vi "Main_updated.vi"() -> ()   [LabVIEW 2016]
uses:
  Spreadsheet filling/Controls/Language Control.ctl
  types/Control_EXIT.ctl
  types/ctrlMainStates.ctl
  types/ctrlMainData.ctl
  Spreadsheet filling/Controls/Information_tab_type.ctl
  types/final data type.ctl
  <vilib>/Utility/miscctls.llb/LVPointTypeDef.ctl
  <vilib>/Utility/config.llb/Read Key (Boolean).vi
  <vilib>/Utility/config.llb/NI_LVConfig.lvlib
panel:
  in  "Exit":T1
  in  "Gas":bool
  out "Volume % Difference":dbl
  out "Progress":dbl(slide) scale=0.0..100.0
  in  "Software Version":string="1.09(US)"
  out "Sample in progress":bool
  out "Collect info done":bool
  in  "Sample method 2":u16(ring) items=["None", "Pulse Input", "Current Input", "Serial Input"]
  out "Mass % Difference":dbl
  in  "Sample \ninterval (S)":dbl=30.0
  in  "Language":T2
  in  "Collect info":bool
  in  "Export report":bool
  in  "Reset table":bool
  in  "Setpoint \n(kg/min)":dbl
  out "Data table":string[][](table)
  in  "Sample method 1":u16(ring) items=["None", "Pulse Input", "Current Input", "Serial Input"]
  in  "Begin pulse sample":bool
  in  "Transfer Data":bool
  in  "Run #":u16
  # "Flow Lifecycle Calibration Services"
  # "Mass\n(UUT)"
  # "Mass\n(Master)"
  # "Mass \n% diff"
  # "Volume\n(UUT)"
  # "Volume\n(Master)"
  # "Setpoint"
  # "Run"
  # "Select an input type"
  # "Select an input type"
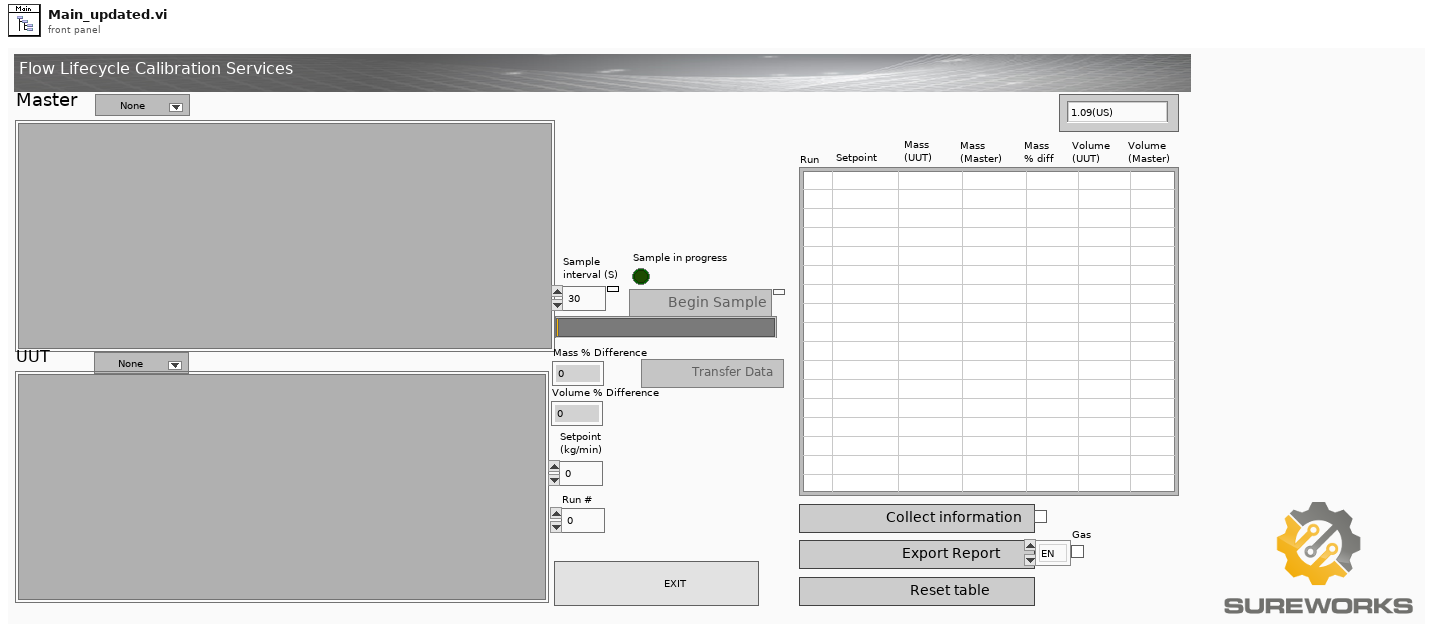
[diagram p1: front panel]
types:
  T1 = typedef "Control_EXIT.ctl" = bool
  T2 = typedef "Language Control.ctl" = enum16{"EN", "ES", "FR", "RU"}
  T3 = typedef "ctrlMainData.ctl" = cluster{"HART ports":refnum<visa-resource-name>[], "485 ports":refnum<visa-resource-name>[], "Byte order":enum16{"0-1-2-3", "2-3-0-1", "1-0-3-2", "3-2-1-0"}, "Information":T4, "Base path":path, "MasterVIRef":refnum<vi>, "UUTVIRef":refnum<vi>, "VIList":string[], "Collect info done":bool, "LeaveExcelOpen":bool, "Sample complete":bool, "Final data":T5, "StartTime":timestamp}
  T4 = typedef "Information_tab_type.ctl" = cluster{"Test Date and Time, 1":string, "Test Comments,3":string, "Sensor Serial Number,6":string, "Sensor Model,7":string, "Size,8":string, "Material,9":string, "Press rating, 10":string, "Temp rating, 11":string, "FCF, 14":string, "D1, 15":string, "D2, 16":string, "K1, 17":string, "K2, 18":string, "FD, 19":string, "Density Temp Coeff, 20":string, "Transmitter Serial Number,23":string, "Transmitter Model Number,24":string, "Mass Flow Units, 25":string, "Density Units, 26":string, "Temperature Units, 27":string, "Mass Flow Cutoff, 28":string, "Mass Flow Damping, 29":string, "Flow Direction, 30":string, "Frequency Flow Rate, 31":string, "Frequency Span, 32":string, "Flow Accuracy, 35":string, "Flow Repeatability, 36":string, "Zero Stability, 37":string, "Density Accuracy, 38":string, "Density Repeatability, 39":string, "Nomincal Flow Rate, 41":string, "Meter Zero, 43":string, "Status, 45":string, "Customer name, 46":string, "Customer address, 47":string, "Sales order number, 48":string, "Technician Name, 49":string, "ref meter, 50":string, "product code,51":string, "fluid,52":string, "fluid temp,53":string}
  T5 = typedef "final data type.ctl" = cluster{"Master final data":cluster{"Mass total":dbl, "Volume total":dbl, "Density mean":dbl}, "UUT final data":cluster{"Mass total":dbl, "Volume total":dbl, "Density mean":dbl}}
  T6 = typedef "ctrlMainStates.ctl" = enum16{"WaitforEvents", "Init", "Close", "SampleStarted", "SampleComplete", "TransferData", "UpdateSampleMethod1", "UpdateSampleMethod2", "ExportReport", "CollectInfo", "ResetTable", "BeginPulseSample"}
  T7 = enum8{"Enabled", "Disabled", "Disabled and Grayed Out"}
  T8 = typedef "LVPointTypeDef.ctl" = cluster{"Horizontal":i16, "Vertical":i16}
  T9 = typedef "NI_LVConfig.lvlib/Config Data RefNum.ctl" = refnum<k1>
  T10 = enum16{"0-1-2-3", "2-3-0-1", "1-0-3-2", "3-2-1-0"}
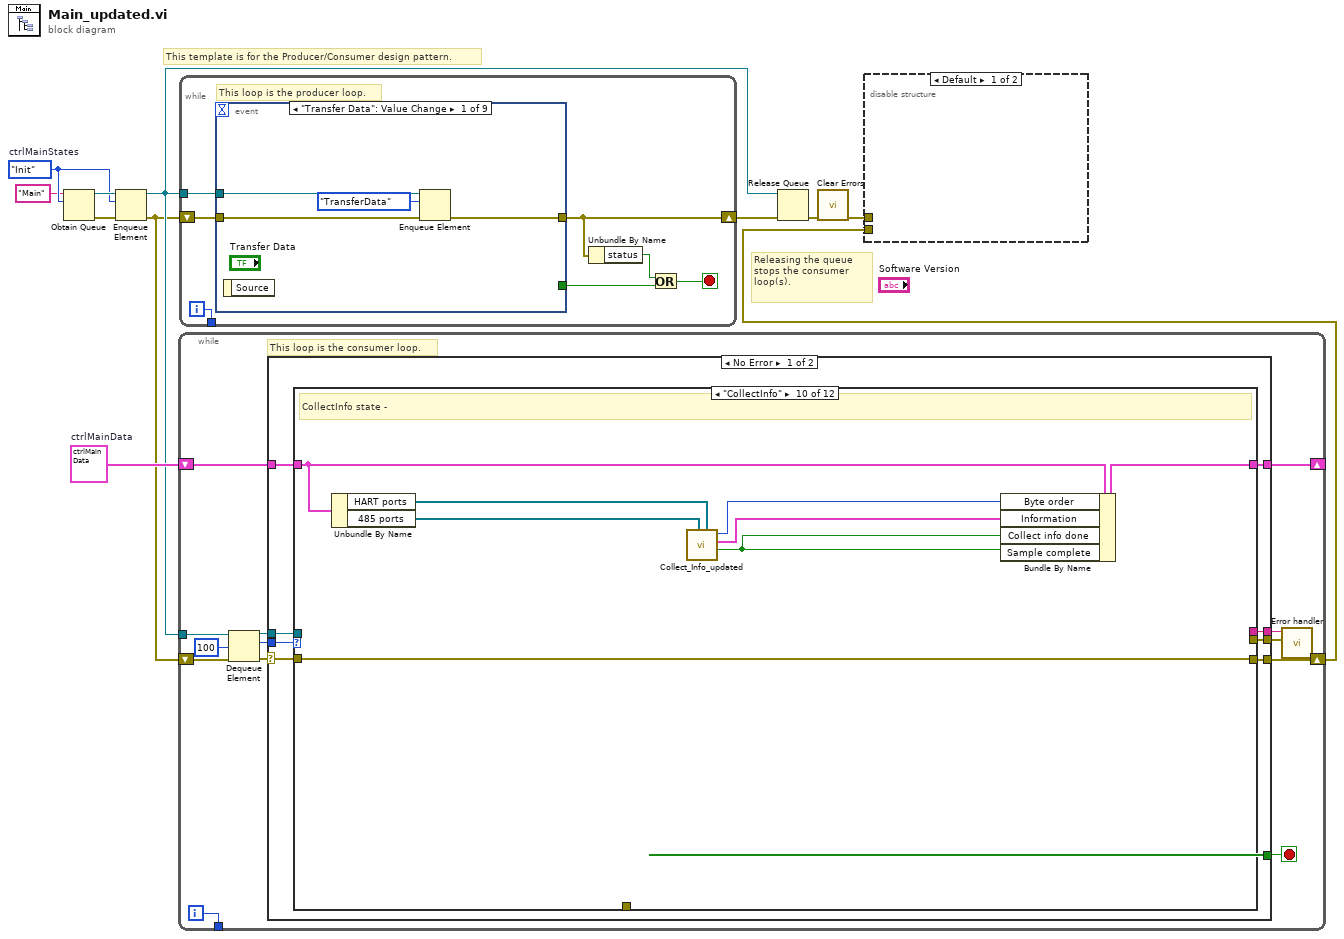
[diagram p0: block diagram]
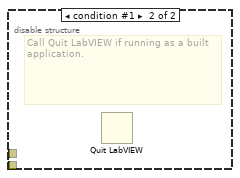
[diagram p2: hidden frame]
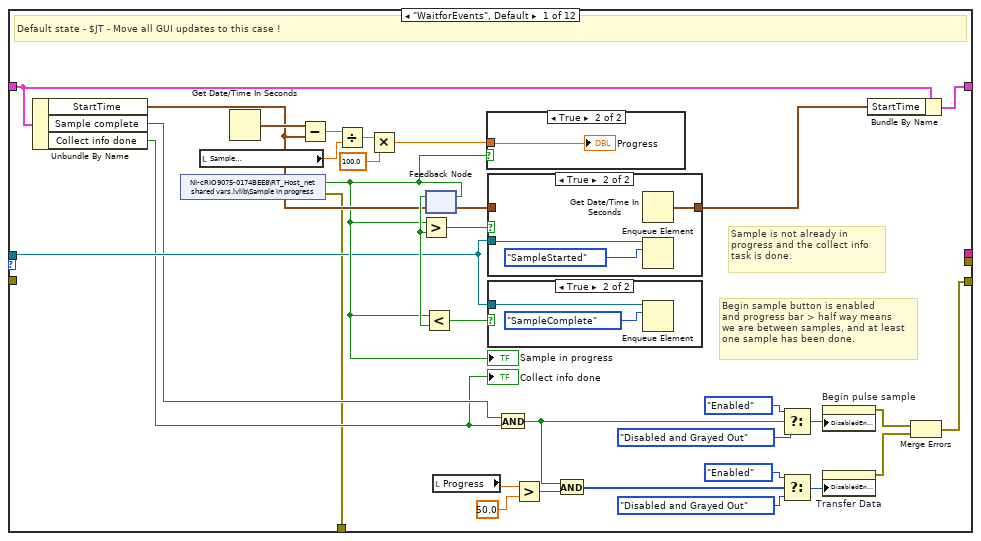
[diagram p3: hidden frame]
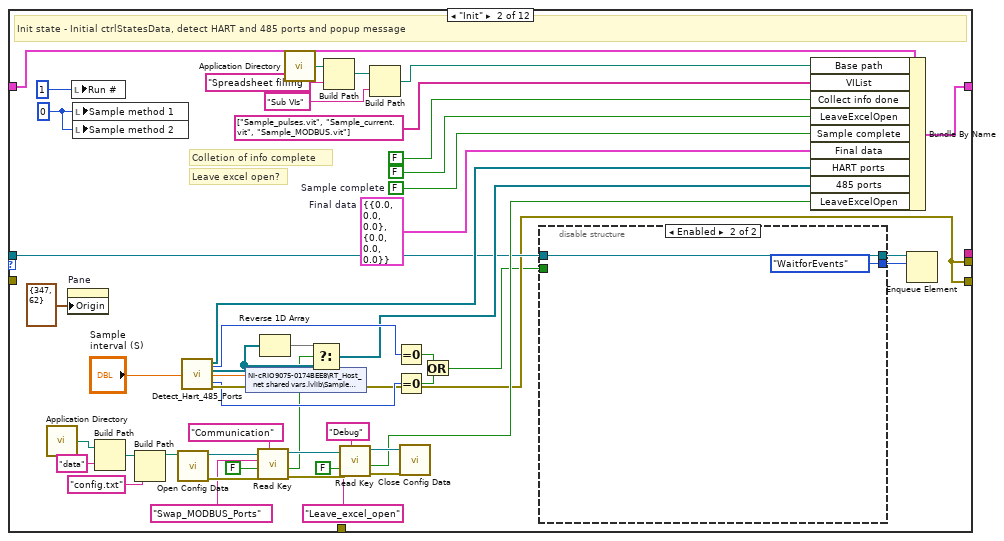
[diagram p7: hidden frame]
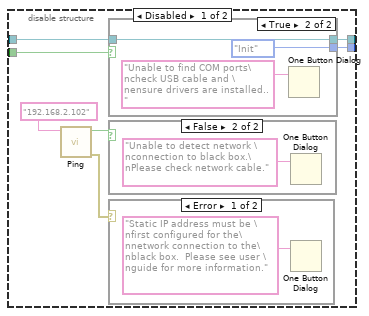
[diagram p8: hidden frame]
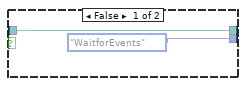
[diagram p9: hidden frame]
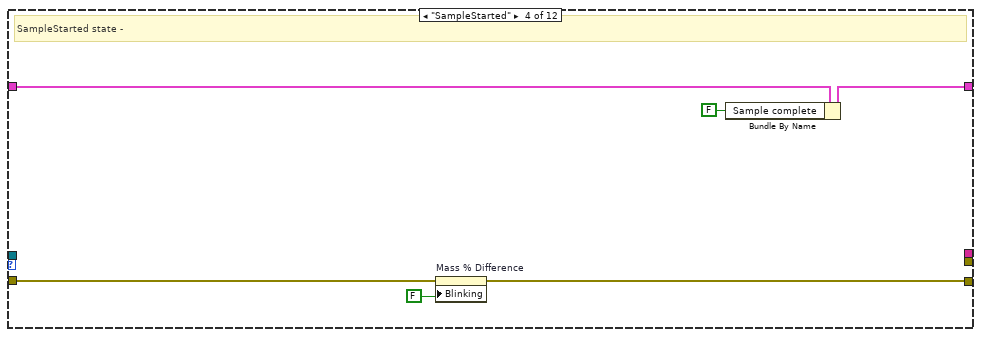
[diagram p13: hidden frame]
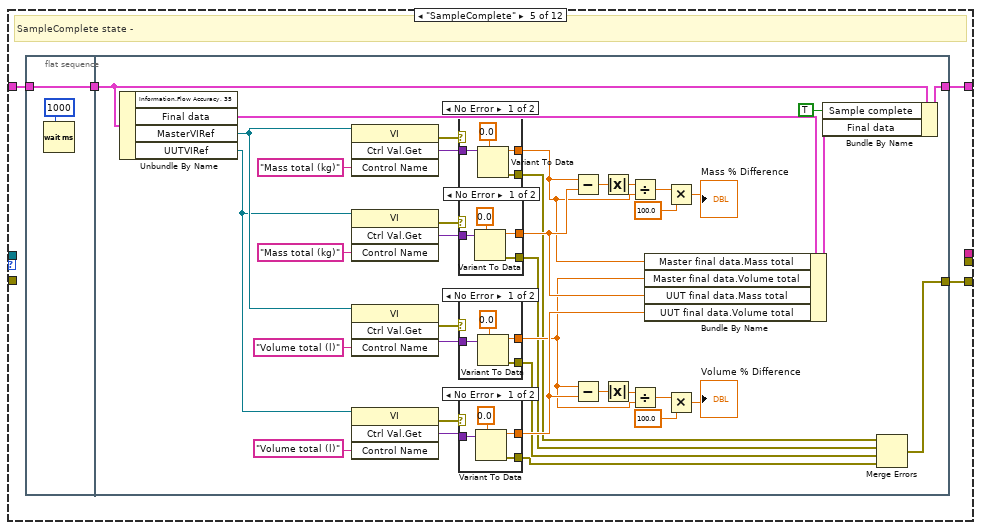
[diagram p14: hidden frame]
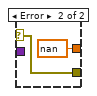
[diagram p15: hidden frame]
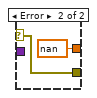
[diagram p16: hidden frame]
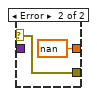
[diagram p17: hidden frame]
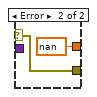
[diagram p18: hidden frame]
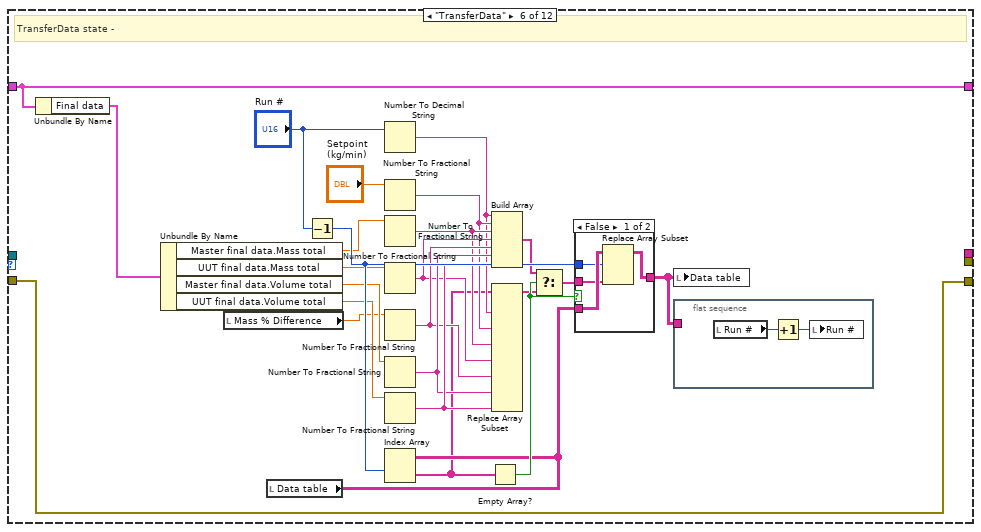
[diagram p19: hidden frame]
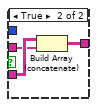
[diagram p20: hidden frame]
diagram:
  w11 = T3 {"HART ports"=[], "485 ports"=[], "Byte order"=enum."0-1-2-3", "Information"={"Test Date and Time, 1"="", "Test Comments,3"="", "Sensor Serial Number,6"="", "Sensor Model,7"="", "Size,8"="", "Material,9"="", "Press rating, 10"="", "Temp rating, 11"="", "FCF, 14"="", "D1, 15"="", "D2, 16"="", "K1, 17"="", "K2, 18"="", "FD, 19"="", "Density Temp Coeff, 20"="", "Transmitter Serial Number,23"="", "Transmitter Model Number,24"="", "Mass Flow Units, 25"="", "Density Units, 26"="", "Temperature Units, 27"="", "Mass Flow Cutoff, 28"="", "Mass Flow Damping, 29"="", "Flow Direction, 30"="", "Frequency Flow Rate, 31"="", "Frequency Span, 32"="", "Flow Accuracy, 35"="", "Flow Repeatability, 36"="", "Zero Stability, 37"="", "Density Accuracy, 38"="", "Density Repeatability, 39"="", "Nomincal Flow Rate, 41"="", "Meter Zero, 43"="", "Status, 45"="", "Customer name, 46"="", "Customer address, 47"="", "Sales order number, 48"="", "Technician Name, 49"="", "ref meter, 50"="", "product code,51"="", "fluid,52"="", "fluid temp,53"=""}, "Base path"=path "", "MasterVIRef"=refnum, "UUTVIRef"=refnum, "VIList"=[], "Collect info done"=FALSE, "LeaveExcelOpen"=FALSE, "Sample complete"=FALSE, "Final data"={"Master final data"={"Mass total"=0.0, "Volume total"=0.0, "Density mean"=0.0}, "UUT final data"={"Mass total"=0.0, "Volume total"=0.0, "Density mean"=0.0}}, "StartTime"=timestamp(0 s since 1904-01-01)}  # ctrlMainData
  w8 = ctrlMainStates."Init"  # ctrlMainStates
  # "This template is for the Producer/Consumer design pattern."
  # "Releasing the queue stops the consumer loop(s)."
  n1 = Obtain Queue(name (unnamed)="Main", element data type=w8) -> (queue out=w10:refnum<queue>, error out=w4:errorcluster)  [unwired: 3 in, 1 out]
  n2 = Enqueue Element(queue=w10, element=w8, error in (no error)=w4) -> (queue out=w9:refnum<queue>, error out=w3:errorcluster)  [unwired: 1 in, 1 out]
  n3 = while {
    tunnel: w9 -> [w24]
    shift-right: [w18] -> _
    shift-left: w11 -> [w20]
    shift-right: [w13] -> w1
    shift-left: w3 -> [w15]
    tunnel: [w12] -> _
    i -> [w12]
    stop <- w21 stop-if-true
    # "This loop is the consumer loop."
    n4 = Dequeue Element(queue=w24, timeout in ms (-1)=100, error in (no error)=w15) -> (queue out=w17:refnum<queue>, element=w22:T6, error out=w23:errorcluster)  [unwired: 1 out]
    n5 = case shown="No Error" w23 {
      selector: w23 -> [w25 w320]
      tunnel: w22 -> [w30 _]
      tunnel: [_ TRUE] -> w21
      tunnel: w20 -> [w31 w321]
      tunnel: [w32 w321] -> w18
      tunnel: w17 -> [w29 _]
      tunnel: [w28 _] -> w14
      tunnel: [w27 _] -> w16
      tunnel: [w26 w319] -> w13
      frame No Error {
        n6 = case shown="\"CollectInfo\"" w30 {
          tunnel: [w55 w109 w138 w141 w148 w215 w250 w263 w281 w299 w305 w318] -> w32
          tunnel: w31 -> [w53 w110 w138 w143 w147 w215 w248 w264 w281 w300 w307 w318]
          tunnel: w29 -> [w50 w77 _ _ _ _ _ _ _ _ _ _]
          tunnel: [_ w74 _ _ _ _ w247 w262 w277 _ _ _] -> w28
          tunnel: [_ _ _ _ _ _ _ _ "Error in PDF path.  Please check that the data output folder exists." ("Error reason") _ _ _] -> w27
          tunnel: [w34 w74 w137 w139 w145 w213 w247 w262 w277 w295 w303 w317] -> w26
          tunnel: w25 -> [_ _ w137 w140 _ w213 _ _ _ w295 w303 w317]
          tunnel: [w33 _ _ _ _ _ _ _ _ _ _ _] -> _
          frame "WaitforEvents", Default {
            # "Begin sample button is enabled\nand progress bar > half way means \nwe are between samples, and at least\none sample has been done."
            # "Sample is not already in\nprogress and the collect info \ntask is done."
            # "Default state - $JT - Move all GUI updates to this case !"
            n7 = Unbundle By Name(w53) -> ("StartTime"=w52:timestamp, "Sample complete"=w46:bool, "Collect info done"=w37:bool)
            "Collect info done" <- w37
            n8 = shared-variable "NI-cRIO9075-0174BEE8\\RT_Host_net shared vars.lvlib\\Sample in progress"() -> (w51:bool, error out=w33:errorcluster)  [unwired: 1 in]
            "Sample in progress" <- w51
            n9 = local read "Sample \ninterval (S)"() -> (w61:dbl)
            n10 = Get Date/Time In Seconds() -> (seconds since 1Jan1904=w59:timestamp)
            n11 = Subtract(x=w59, y=w52) -> (x-y=w60:dbl)
            n12 = Divide(x=w60, y=w61) -> (x/y=w62:dbl)
            n13 = Multiply(x=w62, y=100.0) -> (x*y=w64:dbl)
            n14 = feedback #1() -> (w57:bool)  [unwired: 1 in]
            n15 = Greater?(x=w51, y=w57) -> (0:w56:bool)
            n16 = Less?(x=w51, y=w57) -> (x < y?=w58:bool)
            n17 = feedback-in #1(w51) -> ()
            n18 = local read "Progress"() -> (w41:dbl)
            n19 = case shown="True" w51 {
              tunnel: w64 -> [_ w65]
              frame False {
              }
              frame True {
                "Progress" <- w65
              }
            }
            n20 = case shown="True" w56 {
              tunnel: w50 -> [_ w69]
              tunnel: [w68 w71] -> w54
              tunnel: w52 -> [w68 _]
              frame False {
              }
              frame True {
                n21 = Get Date/Time In Seconds() -> (seconds since 1Jan1904=w71:timestamp)
                n22 = Enqueue Element(queue=w69, element=ctrlMainStates."SampleStarted" ("ctrlStates")) -> ()  [unwired: 2 in, 3 out]
              }
            }
            n23 = case shown="True" w58 {
              tunnel: w50 -> [_ w67]
              frame False {
              }
              frame True {
                n24 = Enqueue Element(queue=w67, element=ctrlMainStates."SampleComplete" ("ctrlStates")) -> ()  [unwired: 2 in, 3 out]
              }
            }
            n25 = And(x=w46, y=w37) -> (x .and. y?=w38:bool)
            n26 = Greater?(x=w41, y=50.0) -> (0:w39:bool)
            n27 = And(x=w38, y=w39) -> (x .and. y?=w42:bool)
            n28 = Select(t=T7."Enabled" ("Disabled"), s=w38, f=T7."Disabled and Grayed Out" ("Disabled")) -> (s? t:f=w47:T7)
            n29 = Select(t=T7."Enabled" ("Disabled"), s=w42, f=T7."Disabled and Grayed Out" ("Disabled")) -> (s? t:f=w43:T7)
            n30 = property on="Begin pulse sample" class="Bool (strict)"("DisabledEnum"=w47) -> (error out=w36:errorcluster)  [unwired: 2 in, 1 out]
            n31 = property on="Transfer Data" class="Bool"("DisabledEnum"=w43) -> (error out=w35:errorcluster)  [unwired: 2 in, 1 out]
            n32 = Bundle By Name(cluster=w53, "StartTime"=w54) -> (w55:T3)
            n33 = Merge Errors(w36, w35) -> (w34:errorcluster)
          }
          frame "Init" {
            w78 = T5 {"Master final data"={"Mass total"=0.0, "Volume total"=0.0, "Density mean"=0.0}, "UUT final data"={"Mass total"=0.0, "Volume total"=0.0, "Density mean"=0.0}}  # Final data
            w79 = FALSE  # Sample complete
            w120 = u16 0 ("Run")
            # "Leave excel open?"
            # "Colletion of info complete"
            # "Init state - Initial ctrlStatesData, detect HART and 485 ports and popup message"
            n34 = call <vilib>:"Application Directory.vi"() -> ("Application Directory"=w104:path)
            n35 = property on="Pane" class="Pane"("Origin"=T8 {"Horizontal"=347, "Vertical"=62}) -> ()  [unwired: 2 in, 2 out]
            n36 = local write "Run #"(u16 1 ("Run #")) -> ()
            n37 = local write "Sample method 1"(w120) -> ()
            n38 = local write "Sample method 2"(w120) -> ()
            n39 = Build Path(base path=w104, name or relative path="data") -> (appended path=w103:path)
            n40 = Build Path(base path=w103, name or relative path="config.txt") -> (appended path=w106:path)
            n41 = call <vilib>:"Open Config Data.vi"("configuration file path"=w106) -> ("error out"=w100:errorcluster, "refnum"=w101:T9)  [unwired: 8 in, 1 out]
            n42 = call "Detect_Hart_485_Ports.vi"() -> ("error out"=w118:errorcluster, "485 Ports"=w112:refnum<visa-resource-name>[], "HART ports"=w108:refnum<visa-resource-name>[], "# 485 ports found"=w114:i32, "# HART ports found"=w115:i32)  [unwired: 6 in, 1 out]
            n43 = shared-variable "NI-cRIO9075-0174BEE8\\RT_Host_net shared vars.lvlib\\Sample period"("Sample \ninterval (S)", error in=w118) -> (error out=w74:errorcluster)
            n44 = call-poly <vilib>:"Read Key.vi"("section"="Communication", "error in (no error)"=w100, "default value"=FALSE, "key"="Swap_MODBUS_Ports", "refnum"=w101) -> ("error out"=w95:errorcluster, "value"=w89:bool, "refnum out"=w96:T9)  [unwired: 3 in, 1 out]
            n45 = Reverse 1D Array(array=w112) -> (reversed array=w113:refnum<visa-resource-name>[])
            n46 = call <vilib>:"Application Directory.vi"() -> ("Application Directory"=w87:path)
            n47 = Select(t=w113, s=w89, f=w112) -> (s? t:f=w107:refnum<visa-resource-name>[])
            n48 = Build Path(base path=w87, name or relative path="Spreadsheet filling") -> (appended path=w85:path)
            n49 = call-poly <vilib>:"Read Key.vi"("section"="Debug", "error in (no error)"=w95, "default value"=FALSE, "key"="Leave_excel_open", "refnum"=w96) -> ("error out"=w94:errorcluster, "value"=w88:bool, "refnum out"=w93:T9)  [unwired: 3 in, 1 out]
            n50 = Build Path(base path=w85, name or relative path="Sub VIs") -> (appended path=w82:path)
            n51 = Equal To 0?(x=w115) -> (x = 0?=w116:bool)
            n52 = Equal To 0?(x=w114) -> (x = 0?=w117:bool)
            n53 = call <vilib>:"Close Config Data.vi"("error in (no error)"=w94, "refnum"=w93) -> ()  [unwired: 8 in, 2 out]
            n54 = Or(x=w116, y=w117) -> (x .or. y?=w73:bool)
            n55 = disable-structure shown="Enabled" {
              disable-tunnel: w77 -> [w124 w136]
              disable-tunnel: [w123 w136] -> w76
              disable-tunnel: [w122 ctrlMainStates."WaitforEvents" ("element")] -> w75
              disable-tunnel: w73 -> [w121 _]
              frame Disabled {
                n56 = call "Ping.vi"("Host IP Address"="192.168.2.102") -> ("error out"=w127:errorcluster, "success"=w126:bool)  [unwired: 8 in, 1 out]
                n57 = case shown="True" w121 {
                  tunnel: w124 -> [w129 w131]
                  tunnel: [w129 w131] -> w123
                  tunnel: [ctrlMainStates."WaitforEvents" ("element") ctrlMainStates."Init" ("element")] -> w122
                  frame False {
                  }
                  frame True {
                    n58 = One Button Dialog(message="Unable to find COM ports\ncheck USB cable and \nensure drivers are installed..") -> ()  [unwired: 1 in, 1 out]
                  }
                }
                n59 = case shown="False" w126 {
                  frame True {
                  }
                  frame False {
                    n60 = One Button Dialog(message="Unable to detect network \nconnection to black box.\nPlease check network cable.") -> ()  [unwired: 1 in, 1 out]
                  }
                }
                n61 = case shown="Error" w127 {
                  frame Error {
                    n62 = One Button Dialog(message="Static IP address must be \nfirst configured for the\nnetwork connection to the\nblack box.  Please see user \nguide for more information.") -> ()  [unwired: 1 in, 1 out]
                  }
                  frame No Error {
                  }
                }
              }
              frame Enabled {
              }
            }
            n63 = Bundle By Name(cluster=w110, "Base path"=w82, "VIList"=string[] ["Sample_pulses.vit", "Sample_current.vit", "Sample_MODBUS.vit"], "Collect info done"=FALSE, "LeaveExcelOpen"=FALSE ("Collect info done"), "Sample complete"=w79, "Final data"=w78, "HART ports"=w108, "485 ports"=w107, "LeaveExcelOpen"=w88) -> (w109:T3)
            n64 = Enqueue Element(queue=w76, element=w75) -> ()  [unwired: 2 in, 3 out]
          }
          frame "Close" {
            # "Close state -"
          }
          frame "SampleStarted" {
            # "SampleStarted state -"
            n65 = property on="Mass % Difference" class="DigNum (strict)"(error in=w140, "Blinking"=FALSE) -> (error out=w139:errorcluster)  [unwired: 1 in, 1 out]
            n66 = Bundle By Name(cluster=w143, "Sample complete"=FALSE) -> (w141:T3)
          }
          frame "SampleComplete" {
            # "SampleComplete state -"
            n67 = flat-sequence {
              tunnel: w147 -> [w150]
              tunnel: [w150] -> w146
              tunnel: [w187] -> w148
              tunnel: w146 -> [w161]
              tunnel: [w151] -> w145
              frame #0 {
                n68 = Wait (ms)(milliseconds to wait=u32 1000) -> ()  [unwired: 1 out]
              }
              frame #1 {
                n69 = Unbundle By Name(w161) -> ("Final data"=w158:T5, "MasterVIRef"=w160:refnum<vi>, "UUTVIRef"=w159:refnum<vi>)  [unwired: 1 out]
                n70 = invoke class="VI" method="Ctrl Val.Get"(reference=w160, "Control Name"="Mass total (kg)") -> (error out=w162:errorcluster, "Get Control Value Variant"=w163:variant)  [unwired: 2 in, 2 out]
                n71 = invoke class="VI" method="Ctrl Val.Get"(reference=w159, "Control Name"="Mass total (kg)") -> (error out=w165:errorcluster, "Get Control Value Variant"=w166:variant)  [unwired: 2 in, 2 out]
                n72 = invoke class="VI" method="Ctrl Val.Get"(reference=w160, "Control Name"="Volume total (l)") -> (error out=w174:errorcluster, "Get Control Value Variant"=w175:variant)  [unwired: 2 in, 2 out]
                n73 = invoke class="VI" method="Ctrl Val.Get"(reference=w159, "Control Name"="Volume total (l)") -> (error out=w177:errorcluster, "Get Control Value Variant"=w176:variant)  [unwired: 2 in, 2 out]
                n74 = case shown="No Error" w162 {
                  selector: w162 -> [_ w205]
                  tunnel: w163 -> [w204 _]
                  tunnel: [w202 nan ("Mass total")] -> w184
                  tunnel: [w201 w205] -> w155
                  frame No Error {
                    n75 = Variant To Data(type=0.0 ("Mass total"), Variant=w204) -> (data=w202:dbl, error out=w201:errorcluster)  [unwired: 1 in]
                  }
                  frame Error {
                  }
                }
                n76 = case shown="No Error" w165 {
                  selector: w165 -> [_ w211]
                  tunnel: w166 -> [w210 _]
                  tunnel: [w208 nan ("Mass total")] -> w185
                  tunnel: [w207 w211] -> w154
                  frame No Error {
                    n77 = Variant To Data(type=0.0 ("Mass total"), Variant=w210) -> (data=w208:dbl, error out=w207:errorcluster)  [unwired: 1 in]
                  }
                  frame Error {
                  }
                }
                n78 = case shown="No Error" w174 {
                  selector: w174 -> [_ w199]
                  tunnel: w175 -> [w198 _]
                  tunnel: [w196 nan ("Mass total")] -> w156
                  tunnel: [w195 w199] -> w153
                  frame No Error {
                    n79 = Variant To Data(type=0.0 ("Mass total"), Variant=w198) -> (data=w196:dbl, error out=w195:errorcluster)  [unwired: 1 in]
                  }
                  frame Error {
                  }
                }
                n80 = case shown="No Error" w177 {
                  selector: w177 -> [_ w193]
                  tunnel: w176 -> [w192 _]
                  tunnel: [w190 nan ("Mass total")] -> w186
                  tunnel: [w189 w193] -> w152
                  frame No Error {
                    n81 = Variant To Data(type=0.0 ("Mass total"), Variant=w192) -> (data=w190:dbl, error out=w189:errorcluster)  [unwired: 1 in]
                  }
                  frame Error {
                  }
                }
                n82 = Subtract(x=w184, y=w185) -> (x-y=w170:dbl)
                n83 = Subtract(x=w156, y=w186) -> (x-y=w180:dbl)
                n84 = Absolute Value(x=w170) -> (abs(x)=w171:dbl)
                n85 = Absolute Value(x=w180) -> (abs(x)=w179:dbl)
                n86 = Divide(x=w171, y=w184) -> (x/y=w168:dbl)
                n87 = Divide(x=w179, y=w156) -> (x/y=w182:dbl)
                n88 = Bundle By Name(cluster=w158, "Master final data.Mass total"=w184, "Master final data.Volume total"=w156, "UUT final data.Mass total"=w185, "UUT final data.Volume total"=w186) -> (w157:T5)
                n89 = Multiply(x=w168, y=100.0) -> (x*y=→"Mass % Difference":dbl)
                n90 = Multiply(x=w182, y=100.0) -> (x*y=→"Volume % Difference":dbl)
                n91 = Bundle By Name(cluster=w161, "Sample complete"=TRUE, "Final data"=w157) -> (w187:T3)
                n92 = Merge Errors(w155, w154, w153, w152) -> (w151:errorcluster)
              }
            }
          }
          frame "TransferData" {
            # "TransferData state -"
            n93 = Unbundle By Name(w215) -> ("Final data"=w214:T5)
            n94 = Unbundle By Name(w214) -> ("Master final data.Mass total"=w233:dbl, "UUT final data.Mass total"=w234:dbl, "Master final data.Volume total"=w235:dbl, "UUT final data.Volume total"=w236:dbl)
            n95 = local read "Mass % Difference"() -> (w229:dbl)
            n96 = local read "Data table"() -> (w224:string[][])
            n97 = Decrement(x="Run #") -> (x-1=w237:u16)
            n98 = Number To Decimal String(number="Run #") -> (decimal integer string=w218:string)  [unwired: 1 in]
            n99 = Number To Fractional String(number="Setpoint \n(kg/min)") -> (F-format string=w219:string)  [unwired: 3 in]
            n100 = Number To Fractional String(number=w233) -> (F-format string=w220:string)  [unwired: 3 in]
            n101 = Number To Fractional String(number=w234) -> (F-format string=w228:string)  [unwired: 3 in]
            n102 = Number To Fractional String(number=w229) -> (F-format string=w230:string)  [unwired: 3 in]
            n103 = Number To Fractional String(number=w235) -> (F-format string=w231:string)  [unwired: 3 in]
            n104 = Number To Fractional String(number=w236) -> (F-format string=w232:string)  [unwired: 3 in]
            n105 = Index Array(array=w224, index (row)=w237) -> (element=w217:string[])  [unwired: 1 in]
            n106 = Empty Array?(array=w217) -> (empty?=w225:bool)
            n107 = Build Array(w218, w219, w220, w228, w230, w231, w232) -> (w222:string[])
            n108 = Replace Array Subset(array=w217, new element #1=w218, new element #2=w219, new element #3=w220, new element #4=w228, new element #5=w230, new element #6=w231, new element #7=w232) -> (w221:string[])  [unwired: 7 in]
            n109 = Select(t=w222, s=w225, f=w221) -> (s? t:f=w223:string[])
            n110 = case shown="False" w225 {
              tunnel: w224 -> [w243 w246]
              tunnel: [w242 w245] -> w227
              tunnel: w237 -> [w241 _]
              tunnel: w223 -> [w240 w244]
              frame False {
                n111 = Replace Array Subset(array=w243, new element=w240, index (row)=w241) -> (w242:string[][])  [unwired: 1 in]
              }
              frame True {
                n112 = Build Array (concatenate)(w246, w244) -> (w245:string[][])
              }
            }
            n113 = local write "Data table"(w227) -> ()
            n114 = flat-sequence {
              tunnel: w227 -> [_]
              frame #0 {
                n115 = local read "Run #"() -> (w239:u16)
                n116 = Increment(x=w239) -> (x+1=w238:u16)
                n117 = local write "Run #"(w238) -> ()
              }
            }
          }
          frame "UpdateSampleMethod1" {
            # "UpdateSampleMethod1 state - UUT's sample method has changed, update the ref."
            n118 = Unbundle By Name(w248) -> ("Base path"=w252:path, "VIList"=w251:string[], "HART ports"=w254:refnum<visa-resource-name>[], "485 ports"=w253:refnum<visa-resource-name>[])  [unwired: 1 out]
            n119 = control-ref of="UUT"() -> (w256:refnum<vi>)
            n120 = Index Array(array=w254, index=1) -> (element=w258:refnum<visa-resource-name>)
            n121 = Index Array(array=w253, index=1) -> (element=w257:refnum<visa-resource-name>)
            n122 = call "Insert_subvi_to_subpanel.vi"("SubVI path"=w252, "HART resource name"=w258, "subpanel ref"=w256, "Input number"=1, "MODBUS resource name"=w257, "Index"="Sample method 1", "Array of VIs to insert"=w251) -> ("error out"=w247:errorcluster, "VI reference out"=w249:refnum<vi>)  [unwired: 3 in]
            n123 = Bundle By Name(cluster=w248, "MasterVIRef"=w249) -> (w250:T3)
          }
          frame "UpdateSampleMethod2" {
            # "UpdateSampleMethod2 state - Mater sample method has changed, update the ref."
            n124 = Unbundle By Name(w264) -> ("Base path"=w269:path, "VIList"=w268:string[], "HART ports"=w265:refnum<visa-resource-name>[], "485 ports"=w266:refnum<visa-resource-name>[])  [unwired: 1 out]
            n125 = control-ref of="Master"() -> (w270:refnum<vi>)
            n126 = Index Array(array=w266, index=0) -> (element=w272:refnum<visa-resource-name>)
            n127 = Index Array(array=w265, index=0) -> (element=w273:refnum<visa-resource-name>)
            n128 = call "Insert_subvi_to_subpanel.vi"("SubVI path"=w269, "HART resource name"=w273, "subpanel ref"=w270, "Input number"=0, "MODBUS resource name"=w272, "Index"="Sample method 2", "Array of VIs to insert"=w268) -> ("error out"=w262:errorcluster, "VI reference out"=w267:refnum<vi>)  [unwired: 3 in]
            n129 = Bundle By Name(cluster=w264, "UUTVIRef"=w267) -> (w263:T3)
          }
          frame "ExportReport" {
            # "ExportReport state -"
            n130 = Unbundle By Name(w281) -> ("Information"=w280:T4, "LeaveExcelOpen"=w279:bool)
            n131 = local read "Data table"() -> (w292:string[][])
            n132 = Not(x=w279) -> (.not. x?=w288:bool)
            n133 = call <vilib>:"Application Directory.vi"() -> ("Application Directory"=w291:path)
            n134 = call "Build Excel File.vi"("close report? (T)"=w288, "Gas"="Gas", "Language"="Language", "Raw data"=w292, "Information"=w280) -> ("error out"=w287:errorcluster, "Excel path"=w285:path, "PDF path out"=w293:path)  [unwired: 3 in, 1 out]
            n135 = Build Path(base path=w291, name or relative path="Test_log.csv") -> (appended path=w289:path)
            n136 = Path To String(path=w285) -> (string=w283:string)
            n137 = call "writelog.vi"("PDF path in"=w293, "data file path"=w289, "Data table"=w292, "Information"=w280) -> ("error out"=w277:errorcluster)  [unwired: 7 in]
            n138 = Concatenate Strings("Error locating the Excel template:" ("Error reason"), w283) -> (w284:string)
            n139 = call "Error handler.vi"("error in"=w287, "Error reason"=w284) -> ()  [unwired: 10 in]
          }
          frame "CollectInfo" {
            # "CollectInfo state -"
            n140 = Unbundle By Name(w300) -> ("HART ports"=w302:refnum<visa-resource-name>[], "485 ports"=w301:refnum<visa-resource-name>[])
            n141 = call "Collect_Info_updated.vi"("HART ports"=w302, "485 Ports"=w301) -> ("Read Completed"=w296:bool, "Information"=w297:T4, "Byte order"=w298:T10)  [unwired: 7 in]
            n142 = Bundle By Name(cluster=w300, "Byte order"=w298, "Information"=w297, "Collect info done"=w296, "Sample complete"=w296) -> (w299:T3)
          }
          frame "ResetTable" {
            # "ResetTable state -"
            n143 = Two Button Dialog(message="Are you sure?", 2:"Yes" ("T button name (\"OK\")")) -> (T button?=w310:bool)  [unwired: 1 in]
            n144 = case shown="True" w310 {
              tunnel: w307 -> [w312 w314]
              tunnel: [w312 w314] -> w306
              tunnel: [w311 FALSE ("Collect info done")] -> w304
              frame False {
                n145 = Unbundle By Name(w312) -> ("LeaveExcelOpen"=w311:bool)
              }
              frame True {
                # "Reset table and run counter"
                # "Reset collection info status"
                n146 = local write "Run #"(u16 1 ("Run")) -> ()
                "Data table" <- string[][] [] ("Raw data")
              }
            }
            n147 = Bundle By Name(cluster=w306, "Collect info done"=w304) -> (w305:T3)
          }
          frame "BeginPulseSample" {
            # "\"BeginPulseSample\" state -"
          }
        }
      }
      frame Error {
        # "Clear errors..."
        # "Return true in any case that should stop the loop."
        n148 = call <vilib>:"Clear Errors.vi"("error in (no error)"=w320) -> ("error out"=w319:errorcluster)  [unwired: 5 in, 1 out]
      }
    }
    n149 = call "Error handler.vi"("error in"=w14, "Error reason"=w16) -> ()  [unwired: 10 in]
  }
  n150 = while {
    tunnel: w9 -> [w329]
    tunnel: [w328] -> _
    shift-right: [w324] -> w2
    shift-left: w3 -> [w327]
    i -> [w328]
    stop <- w325 stop-if-true
    # "This loop is the producer loop."
    n151 = event shown="[0] \"Transfer Data\": Value Change" {
      selector: _ -> [_ _ _ _ _ _ _ _ _]
      dyn-events: _ -> [_ _ _ _ _ _ _ _ _]
      timeout: _ -> [_ _ _ _ _ _ _ _ _]
      tunnel: w329 -> [w333 w337 w341 w345 w349 w353 w357 _ _]
      tunnel: w327 -> [w331 w335 w339 w343 w347 w351 w355 w362 w367]
      tunnel: [w330 w334 w338 w342 w346 w350 w354 w362 w367] -> w324
      tunnel: [_ _ _ _ _ _ _ w359 w363] -> w323
      event "Transfer Data": Value Change {
        n152 = event-data() -> ()  [unwired: 1 in, 1 out]
        n153 = Enqueue Element(queue=w333, element=ctrlMainStates."TransferData", error in (no error)=w331) -> (error out=w330:errorcluster)  [unwired: 1 in, 2 out]
      }
      event "Sample method 1": Value Change {
        n154 = event-data() -> ()  [unwired: 1 in, 1 out]
        n155 = Enqueue Element(queue=w337, element=ctrlMainStates."UpdateSampleMethod1", error in (no error)=w335) -> (error out=w334:errorcluster)  [unwired: 1 in, 2 out]
      }
      event "Sample method 2": Value Change {
        n156 = event-data() -> ()  [unwired: 1 in, 1 out]
        n157 = Enqueue Element(queue=w341, element=ctrlMainStates."UpdateSampleMethod2", error in (no error)=w339) -> (error out=w338:errorcluster)  [unwired: 1 in, 2 out]
      }
      event "Export report": Value Change {
        n158 = event-data() -> ()  [unwired: 1 in, 1 out]
        n159 = Enqueue Element(queue=w345, element=ctrlMainStates."ExportReport", error in (no error)=w343) -> (error out=w342:errorcluster)  [unwired: 1 in, 2 out]
      }
      event "Collect info": Value Change {
        n160 = event-data() -> ()  [unwired: 1 in, 1 out]
        n161 = Enqueue Element(queue=w349, element=ctrlMainStates."CollectInfo", error in (no error)=w347) -> (error out=w346:errorcluster)  [unwired: 1 in, 2 out]
      }
      event "Reset table": Value Change {
        n162 = event-data() -> ()  [unwired: 1 in, 1 out]
        n163 = Enqueue Element(queue=w353, element=ctrlMainStates."ResetTable", error in (no error)=w351) -> (error out=w350:errorcluster)  [unwired: 1 in, 2 out]
      }
      event "Begin pulse sample": Value Change {
        n164 = event-data() -> ()  [unwired: 1 in, 1 out]
        n165 = Enqueue Element(queue=w357, element=ctrlMainStates."BeginPulseSample", error in (no error)=w355) -> (error out=w354:errorcluster)  [unwired: 1 in, 2 out]
      }
      event Panel Close? {
        (unwired) "Cancel" ("F button name (\"Cancel\")")
        n166 = event-data() -> ()  [unwired: 1 in, 1 out]
        n167 = Two Button Dialog(message="Quitting will Abort all running program\nAre you sure you want to exit?", 2:"Quit" ("T button name (\"OK\")")) -> (T button?=w359:bool)  [unwired: 1 in]
        n168 = Not(x=w359) -> (.not. x?=w358:bool)
        n169 = event-data("Discard?"=w358) -> ()  [unwired: 1 in, 1 out]
      }
      event Value Change {
        n170 = event-data() -> ()  [unwired: 1 in, 1 out]
        n171 = Two Button Dialog(message="Quitting will Abort all running program\nAre you sure you want to exit?", 1:"Cancel" ("F button name (\"Cancel\")"), 2:"Quit" ("T button name (\"OK\")")) -> (T button?=w363:bool)
      }
    }
    n172 = Unbundle By Name(w324) -> ("status"=w326:bool)
    n173 = Or(x=w326, y=w323) -> (x .or. y?=w325:bool)
  }
  n174 = Release Queue(queue=w9, error in (no error)=w2) -> (error out=w5:errorcluster)  [unwired: 1 in, 2 out]
  n175 = call <vilib>:"Clear Errors.vi"("error in (no error)"=w5) -> ("error out"=w6:errorcluster)  [unwired: 5 in, 1 out]
  n176 = disable-structure shown="Default" {
    disable-tunnel: w6 -> [_ _]
    disable-tunnel: w1 -> [_ _]
    frame condition #0 (active) {
    }
    frame condition #1 {
      # "Call Quit LabVIEW if running as a built application."
      n177 = Quit LabVIEW() -> ()  [unwired: 1 in]
    }
  }
